vi "On Permission Requested.vi"(8 "error in (no error)":errorcluster, 10 "Data":T2, 11 "WebView2 Event Filter Interface in":refnum<class "WebView2 Event Filter Interface.lvclass">) -> (0 "error out":errorcluster, 2 "Response":T1 {"State" items=["Default", "Allow", "Deny"]})   [LabVIEW 2025, in "WebView2.lvlib" / "WebView2 Event Filter Interface.lvclass"]
uses:
  WebView2 Event Filter Interface.lvclass
  WebView2 Control Object/Permission Requested Event Data.ctl
  WebView2 Control Object/WebView2 Control.lvclass
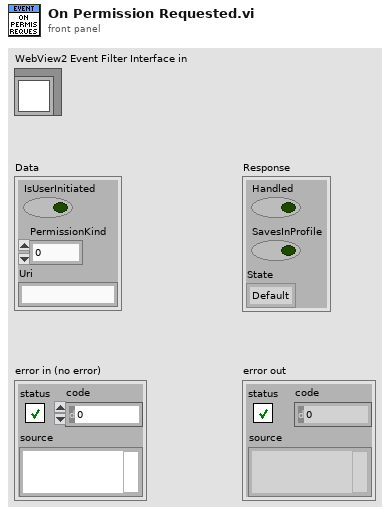
[diagram p1: front panel]
types:
  T1 = cluster{"Handled":bool, "SavesInProfile":bool, "State":i32}
  T2 = typedef "WebView2.lvlib/WebView2 Control.lvclass/Permission Requested Event Data.ctl" = cluster{"IsUserInitiated":bool, "PermissionKind":i32, "Uri":string}
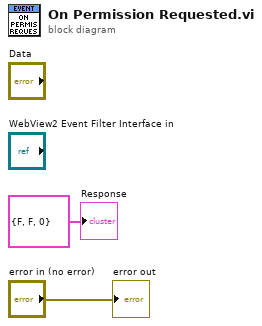
[diagram p0: block diagram]
diagram:
  "error out" <- "error in (no error)"
  "Response" <- T1 {"Handled"=FALSE, "SavesInProfile"=FALSE, "State"=0} ("Response")
